vi "Add Parameter.vi"(8 "error in":errorcluster, 10 "parameter configuration":T1, 11 "label in":refnum<k24>) -> (0 "error out":errorcluster, 2 "new parameter":refnum<k24>, 3 "label out":refnum<k24>)   [LabVIEW 2020, in "AIM_Parameter_ni.lvlib"]
uses:
  AIM_Parameter_ni.lvlib
  C:/Users/Administrator/Desktop/GIT/Ballard-Arinc-429-XML-Generator/Source/Assemblies/Aim_Parameter_ni/bin/Debug/AIM_429_Parameter_ni.dll
  Assemblies/Aim_Parameter_ni/bin/Debug/AIM_429_Parameter_ni.dll
  _tyedefs/parameter_type.ctl
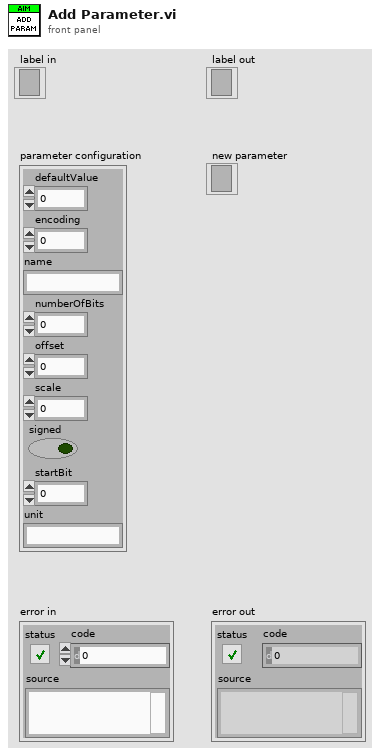
[diagram p1: front panel]
types:
  T1 = typedef "AIM_Parameter_ni.lvlib/parameter_type.ctl" = cluster{"defaultValue":dbl, "encoding":i32, "name":string, "numberOfBits":i32, "offset":dbl, "scale":dbl, "signed":bool, "startBit":i32, "unit":string}
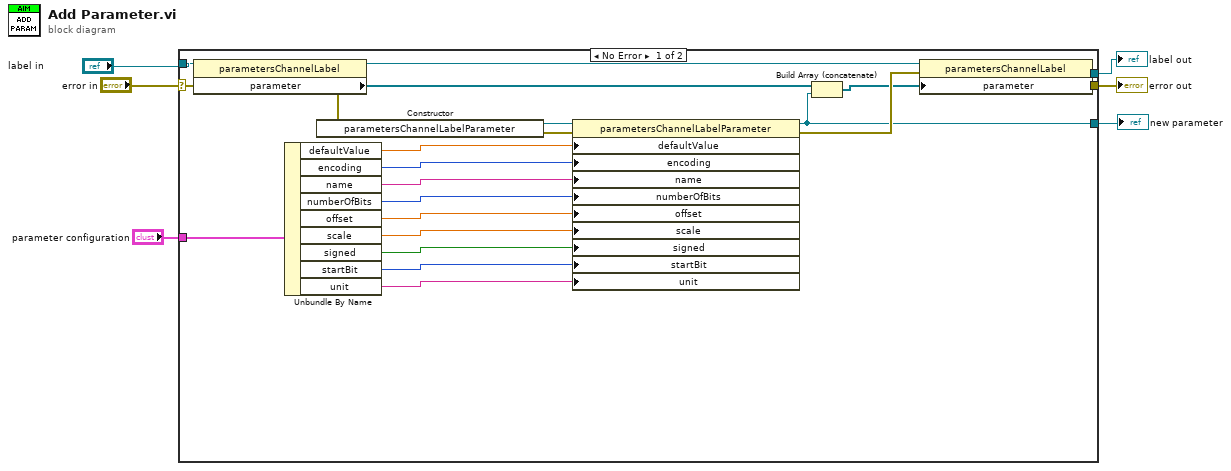
[diagram p0: block diagram]
diagram:
  n1 = case shown="No Error" "error in" {
    selector: "error in" -> [w27 w29]
    tunnel: [w23 w30] -> w6
    tunnel: [w22 w29] -> w5
    tunnel: "label in" -> [w28 w30]
    tunnel: [w8 _] -> w1
    tunnel: "parameter configuration" -> [w18 _]
    frame No Error {
      n2 = property class="parametersChannelLabel"(reference=w28, error in=w27) -> (reference out=w24:refnum<k24>, error out=w25:errorcluster, "parameter"=w26:refnum<k24>[])
      n3 = Unbundle By Name(w18) -> ("defaultValue"=w17:dbl, "encoding"=w16:i32, "name"=w15:string, "numberOfBits"=w14:i32, "offset"=w13:dbl, "scale"=w12:dbl, "signed"=w11:bool, "startBit"=w10:i32, "unit"=w9:string)
      n4 = constructor class="parametersChannelLabelParameter"(error in=w25) -> (reference out=w21:refnum<k24>, error out=w20:errorcluster)  [unwired: 2 in, 1 out]
      n5 = property class="parametersChannelLabelParameter"(reference=w21, error in=w20, "defaultValue"=w17, "encoding"=w16, "name"=w15, "numberOfBits"=w14, "offset"=w13, "scale"=w12, "signed"=w11, "startBit"=w10, "unit"=w9) -> (reference out=w8:refnum<k24>, error out=w19:errorcluster)
      n6 = Build Array (concatenate)(w26, w8) -> (w7:refnum<k24>[])
      n7 = property class="parametersChannelLabel"(reference=w24, error in=w19, "parameter"=w7) -> (reference out=w23:refnum<k24>, error out=w22:errorcluster)
    }
    frame Error {
    }
  }
  "label out" <- w6
  "error out" <- w5
  "new parameter" <- w1
